vi "Display Module - Set Display Order.vi"() -> ()   [LabVIEW 2016]
uses:
  <vilib>/vision/Image Controls.llb/IMAQ Image.ctl
panel:
  in  "IMAQ Display Refs":refnum<vi>[](array[refnum])
  in  "Exit":bool
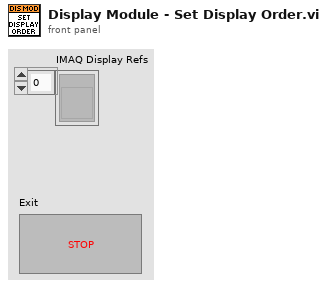
[diagram p1: front panel]
types:
  T1 = typedef "IMAQ Image.ctl" = refnum<image>
  T2 = enum32{"Bad", "Idle", "Run top level", "Running"}
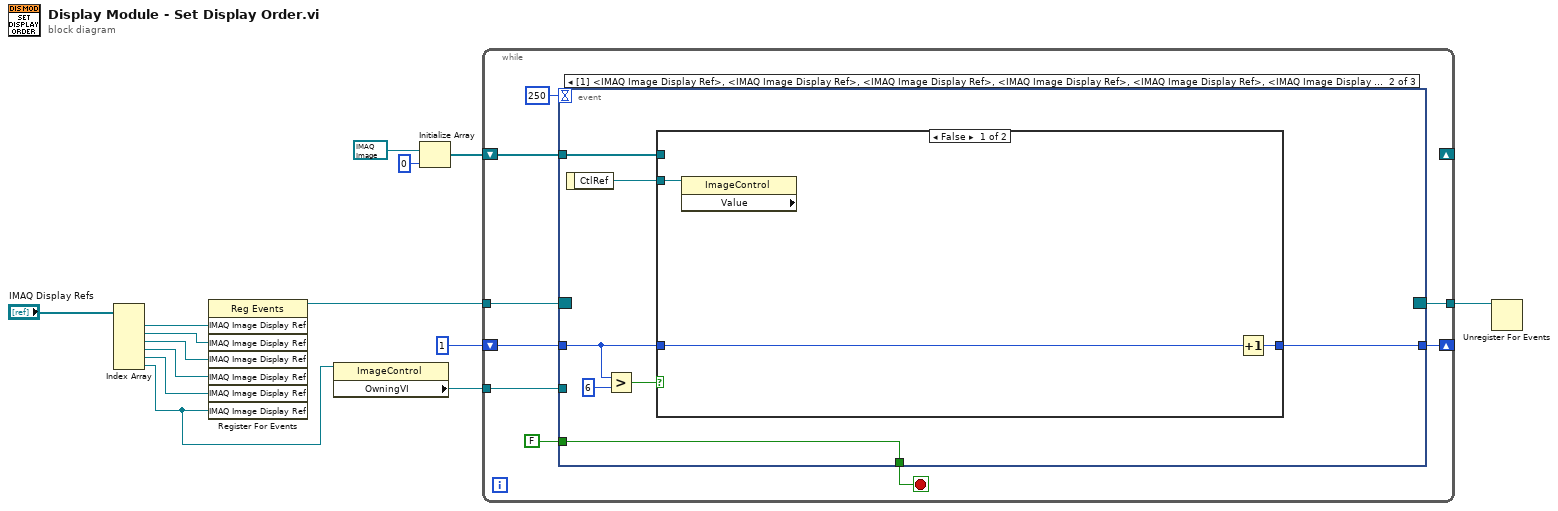
[diagram p0: block diagram]
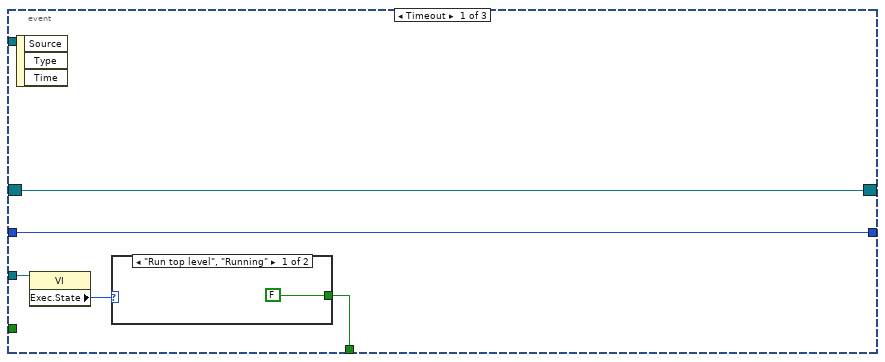
[diagram p2: hidden frame]
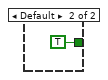
[diagram p3: hidden frame]
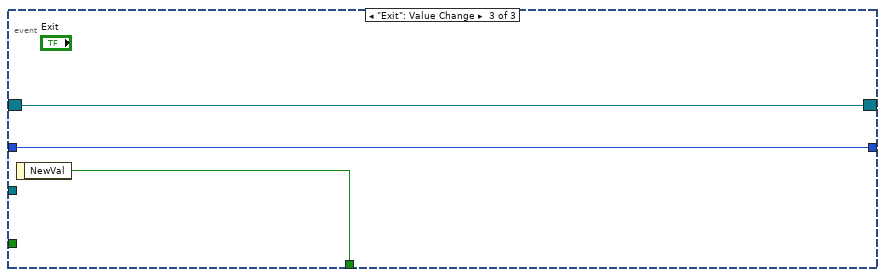
[diagram p5: hidden frame]
diagram:
  n1 = Index Array(array="IMAQ Display Refs") -> (element #1=w9:refnum<vi>, element #2=w13:refnum<vi>, element #3=w10:refnum<vi>, element #4=w11:refnum<vi>, element #5=w12:refnum<vi>, element #6=w5:refnum<vi>)  [unwired: 6 in]
  n2 = register-events(w9, w13, w10, w11, w12, w5) -> (reference out=w8:refnum<event-registration>)  [unwired: 2 in, 1 out]
  n3 = property class="ImageControl"(reference=w5) -> ("OwningVI"=w4:refnum<vi>)  [unwired: 1 in, 2 out]
  n4 = Initialize Array(T1 refnum ("New Image"), 0 ("dimension size")) -> (w1:T1[])
  n5 = while {
    tunnel: w8 -> [w20]
    tunnel: [w19] -> w7
    shift-right: [w17] -> _
    shift-left: 1 -> [w18]
    tunnel: w4 -> [w16]
    shift-right: _ -> [_]
    shift-left: w1 -> [w15]
    stop <- w23 stop-if-true
    n6 = event shown="[1] <IMAQ Image Display Ref>, <IMAQ Image Display Ref>, <IMAQ Image Display Ref>, <IMAQ Image Display Ref>, <IMAQ Image Display Ref>, <IMAQ Image Display Ref>: Mouse Up" {
      selector: w20 -> [w24 _ w43]
      dyn-events: [w24 _ w43] -> w19
      timeout: 250 -> [_ _ _]
      tunnel: [w27 w37 w44] -> w23
      tunnel: FALSE -> [_ w37 _]
      tunnel: w18 -> [w25 w34 w42]
      tunnel: [w25 w32 w42] -> w17
      tunnel: w16 -> [w26 _ _]
      tunnel: w15 -> [_ w31 _]
      event Timeout {
        n7 = event-data() -> ()  [unwired: 1 in, 3 out]
        n8 = property class="VI"(reference=w26) -> ("Exec.State"=w28:T2)  [unwired: 1 in, 2 out]
        n9 = case shown="\"Run top level\", \"Running\"" w28 {
          tunnel: [FALSE TRUE] -> w27
          frame "Run top level", "Running" {
          }
          frame Default {
          }
        }
      }
      event Mouse Up {
        n10 = event-data() -> ("CtlRef"=w33:refnum<vi>)  [unwired: 1 in]
        n11 = Greater?(x=w34, y=6) -> (0:w35:bool)
        n12 = case shown="False" w35 {
          tunnel: w34 -> [w40 w41]
          tunnel: w33 -> [w38 _]
          tunnel: [w39 w41] -> w32
          tunnel: w31 -> [_ _]
          frame False {
            n13 = property class="ImageControl" props=["Value"](reference=w38) -> ()  [unwired: 1 in, 3 out]
            n14 = Increment(x=w40) -> (x+1=w39:i32)
          }
          frame True {
          }
        }
      }
      event "Exit": Value Change {
        n15 = event-data() -> ("NewVal"=w44:bool)  [unwired: 1 in]
      }
    }
  }
  n16 = Unregister For Events(event registration refnum=w7) -> ()  [unwired: 1 in, 1 out]
